vi "FalconHistogram.vi"() -> ()   [LabVIEW 2011]
uses:
  <vilib>/Analysis/NI_AALBase.lvlib
panel:
  out "SNR?":dbl
  out "TotalSum":dbl
  out "Signal":dbl
  out "median (all)":dbl format="%0.2f"
  out "mean (all)":dbl format="%0.2f"
  in  "Plot ...":bool
  in  "ImageBuffer":u32[][](graph)
  in  "GrayLevels":u8[][](graph)
  out "All Image":T1(graph)
  out "Pourtour":T1(graph)
  out "mean":dbl format="%0.2f"
  out "median":dbl format="%0.2f"
  out "output array":u32[](array[numeric])
  out "size(s)":i32[](array[numeric])
  # "GrayLevels"
  # "ImageBuffer"
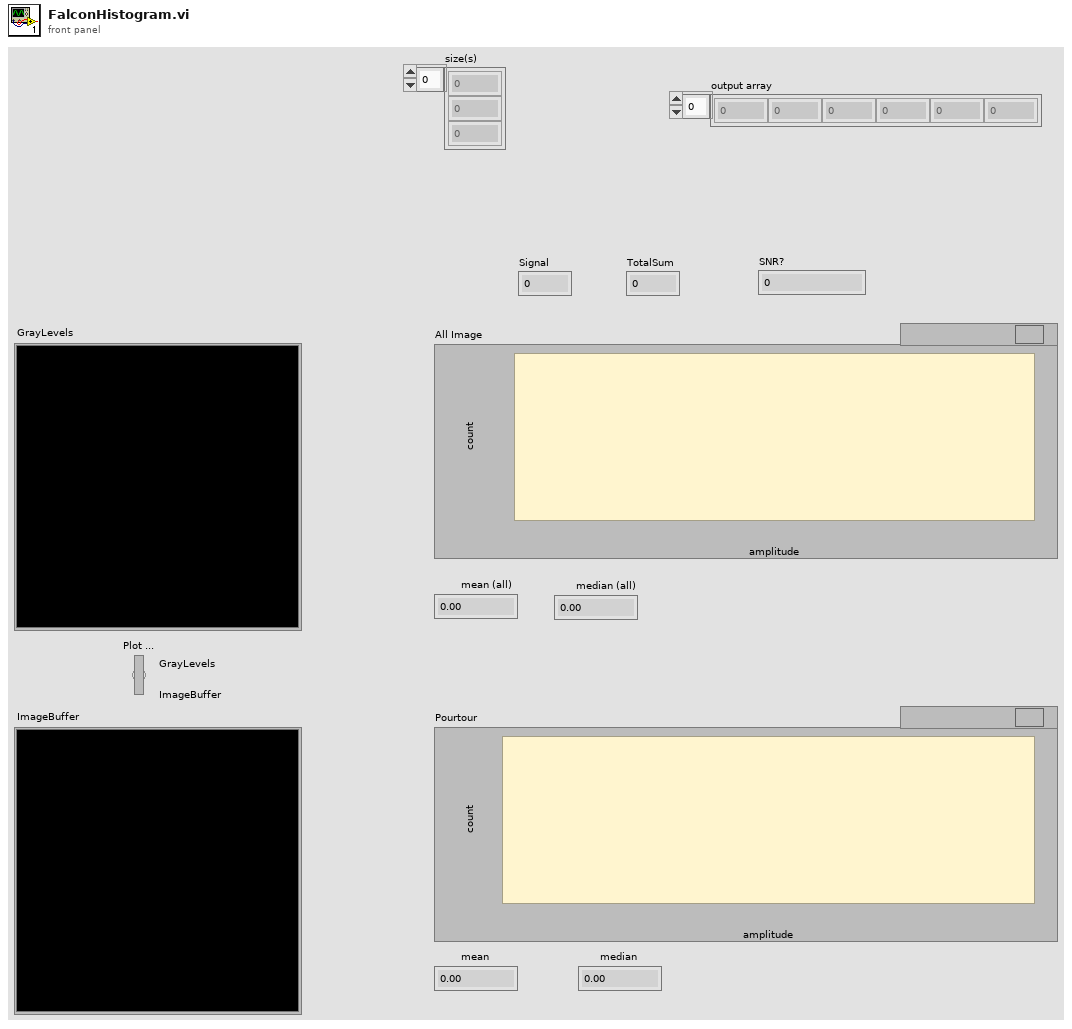
[diagram p1: front panel]
types:
  T1 = cluster{"X Values":dbl[], "Histogram: h(x)":i32[]}
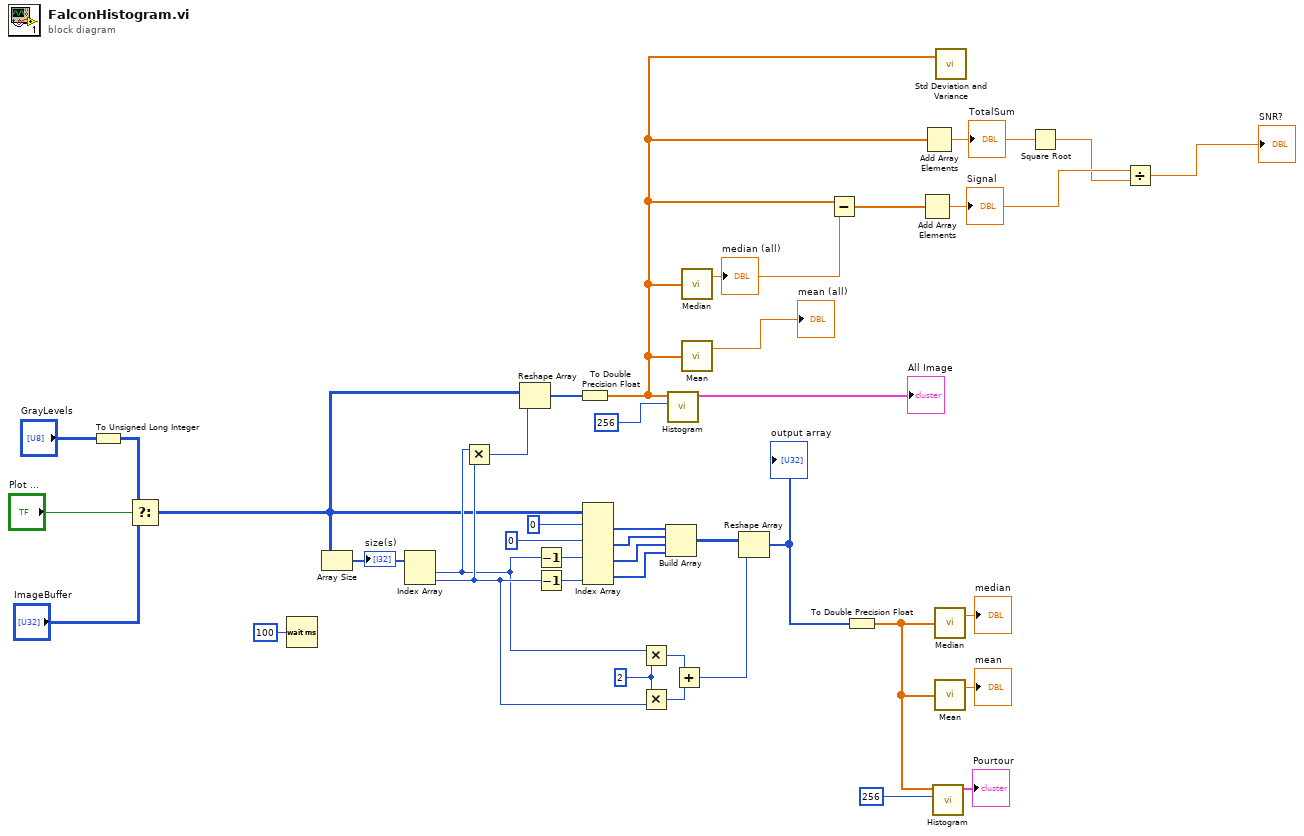
[diagram p0: block diagram]
diagram:
  w25 = 2
  n1 = To Unsigned Long Integer(number="GrayLevels") -> (unsigned 32bit integer=w12:u32[][])
  n2 = Select(t=w12, s="Plot ...", f="ImageBuffer") -> (s? t:f=w10:u32[][])
  n3 = Wait (ms)(milliseconds to wait=u32 100) -> ()  [unwired: 1 out]
  n4 = Array Size(array=w10) -> (size(s)=w40:i32[])
  "size(s)" <- w40
  n5 = Index Array(array=w40) -> (element #1=w19:i32, element #2=w20:i32)  [unwired: 2 in]
  n6 = Multiply(x=w19, y=w20) -> (x*y=w18:i32)
  n7 = Reshape Array(w10, w18) -> (w17:u32[])
  n8 = Decrement(x=w19) -> (x-1=w37:i32)
  n9 = Decrement(x=w20) -> (x-1=w36:i32)
  n10 = To Double Precision Float(number=w17) -> (double precision float=w5:dbl[])
  n11 = Index Array(array=w10, index (row) #1=0 ("index (row)"), index (col) #2=0 ("disabled index (col)"), index (row) #3=w37, index (col) #4=w36) -> (element #1=w34:u32[], element #2=w33:u32[], element #3=w32:u32[], element #4=w35:u32[])  [unwired: 4 in]
  n12 = Multiply(x=w19, y=w25) -> (x*y=w27:i32)
  n13 = Multiply(x=w25, y=w20) -> (x*y=w26:i32)
  n14 = Build Array(w34, w33, w32, w35) -> (w31:u32[][])
  n15 = call <vilib>:"Histogram.vi"("intervals"=256, "X"=w5) -> ("Histogram Graph"=→"All Image":T1)  [unwired: 6 in, 3 out]
  n16 = Add(x=w27, y=w26) -> (x+y=w24:i32)
  n17 = call <vilib>:"Median.vi"("X"=w5) -> ("median"=w7:dbl)  [unwired: 1 out]
  "median (all)" <- w7
  n18 = call <vilib>:"Mean.vi"("X"=w5) -> ("mean"=→"mean (all)":dbl)  [unwired: 1 out]
  n19 = Reshape Array(w31, w24) -> (w30:u32[])
  "output array" <- w30
  n20 = Subtract(x=w5, y=w7) -> (x-y=w6:dbl[])
  n21 = To Double Precision Float(number=w30) -> (double precision float=w23:dbl[])
  n22 = Add Array Elements(numeric array=w6) -> (sum=w4:dbl)
  "Signal" <- w4
  n23 = Add Array Elements(numeric array=w5) -> (sum=w3:dbl)
  "TotalSum" <- w3
  n24 = call <vilib>:"Histogram.vi"("intervals"=256, "X"=w23) -> ("Histogram Graph"=→"Pourtour":T1)  [unwired: 6 in, 3 out]
  n25 = call <vilib>:"Median.vi"("X"=w23) -> ("median"=→"median":dbl)  [unwired: 1 out]
  n26 = call <vilib>:"Mean.vi"("X"=w23) -> ("mean"=→"mean":dbl)  [unwired: 1 out]
  n27 = call <vilib>:"Std Deviation and Variance.vi"("X"=w5) -> ()  [unwired: 1 in, 3 out]
  n28 = Square Root(x=w3) -> (sqrt(x)=w2:dbl)
  n29 = Divide(x=w4, y=w2) -> (x/y=→"SNR?":dbl)
